vi "Config Drive Module Get-Set.vi"(4 "Start with Default":bool, 6 "Get(f) Set(t)":bool, 7 "Set Drive Config":T1={"Drive HW Ver"=0, "SparkMax Output"={"Idle Mode"=enum."Coast", "Ramp Rate (S)"=1.0}, "Slot 0 CL"={"Gains"={"P"=0.1, "I"=0.0, "D"=0.0, "F"=0.0}, "I Zone"=0.0, "Peak Out -1 0 1"={"High"=0.0, "Low"=0.0}, "Max I Accu"=0.0}, "Slot 0 SM"={"Max Velocity"=0.0, "Max Acceleration"=0.0, "Allowed CL Error"=0.0, "Min Velocity Output"=0.0}} {"Slot 0 CL"."Gains"."F" format="%#.8f"; "Slot 0 CL"."Gains"."D" format="%#.8f"; "Slot 0 CL"."Gains"."I" format="%#.8f"; "Slot 0 CL"."Gains"."P" format="%#.8f"; "Slot 0 CL"."Peak Out -1 0 1"."Low" format="%#.8f"; "Slot 0 CL"."Peak Out -1 0 1"."High" format="%#.8f"}, 8 "Error":errorcluster, 11 "Drive Refs":T8) -> (0 "Error Out":errorcluster, 3 "Drive Refs Out":T8, 5 "Drive Config Out":T1={"Drive HW Ver"=0, "SparkMax Output"={"Idle Mode"=enum."Coast", "Ramp Rate (S)"=1.0}, "Slot 0 CL"={"Gains"={"P"=0.1, "I"=0.0, "D"=0.0, "F"=0.0}, "I Zone"=0.0, "Peak Out -1 0 1"={"High"=0.0, "Low"=0.0}, "Max I Accu"=0.0}, "Slot 0 SM"={"Max Velocity"=0.0, "Max Acceleration"=0.0, "Allowed CL Error"=0.0, "Min Velocity Output"=0.0}} {"Slot 0 CL"."Gains"."F" format="%#.8f"; "Slot 0 CL"."Gains"."D" format="%#.8f"; "Slot 0 CL"."Gains"."I" format="%#.8f"; "Slot 0 CL"."Gains"."P" format="%#.8f"; "Slot 0 CL"."Peak Out -1 0 1"."Low" format="%#.8f"; "Slot 0 CL"."Peak Out -1 0 1"."High" format="%#.8f"})   [LabVIEW 2023, in "Swerve AM_ACT.lvlib"]
uses:
  Swerve AM_ACT.lvlib
  t-shirt-robot/T-Shirt Robot LV 2020/roboRIO Code/Systems/SwerveDrive AM/Cluster_Config Drive HW Values.ctl
  Shared Code/TypeDefs/Cluster_Config Spark Max Motor Output.ctl
  <vilib>/Rock Robotics/WPI/ThirdParty/REV Robotics/REVLib/Typedef/Spark MAX Idle Mode.ctl
  Shared Code/TypeDefs/Cluster_Spark MAX SLOT PID Config.ctl
  Shared Code/TypeDefs/Cluster_PID Gains.ctl
  Shared Code/TypeDefs/Cluster_High-Low.ctl
  Shared Code/TypeDefs/Cluster_SparkMax Smart Motion Parameters.ctl
  <vilib>/Rock Robotics/WPI/MotorControl/WPI_MotorControlDeviceRef.ctl
  <vilib>/Rock Robotics/WPI/MotorControl/WPI_MotorControlType.ctl
  <vilib>/Rock Robotics/SystemInterfaces/DIO/FPGA_DIOPWMChannel.ctl
  <vilib>/Rock Robotics/WPI/PWM/WPI_PWMDeadband.ctl
  <vilib>/Rock Robotics/SystemInterfaces/DIO/FPGA_DIOChannel.ctl
  <vilib>/Utility/error.llb/Trim Whitespace One-Sided.vi
  <vilib>/Utility/Data Type/NI_Data Type.lvlib
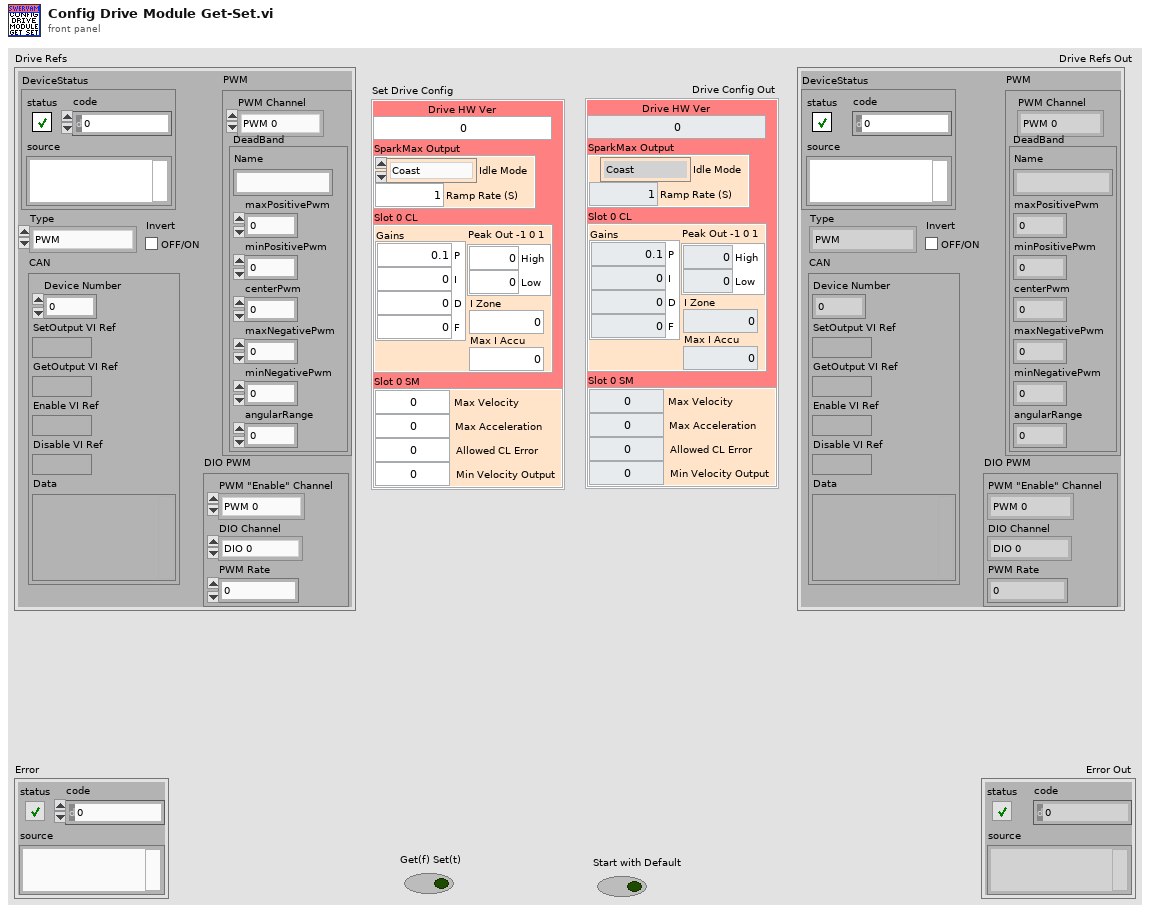
[diagram p1: front panel]
types:
  T1 = typedef "Swerve AM_ACT.lvlib/Cluster_Config Drive HW Values.ctl" = cluster{"Drive HW Ver":u64, "SparkMax Output":T2, "Slot 0 CL":T4, "Slot 0 SM":T7}
  T2 = typedef "Cluster_Config Spark Max Motor Output.ctl" = cluster{"Idle Mode":T3, "Ramp Rate (S)":dbl}
  T3 = typedef "Spark MAX Idle Mode.ctl" = enum16{"Coast", "Brake"}
  T4 = typedef "Cluster_Spark MAX SLOT PID Config.ctl" = cluster{"Gains":T5, "I Zone":dbl, "Peak Out -1 0 1":T6, "Max I Accu":dbl}
  T5 = typedef "Cluster_PID Gains.ctl" = cluster{"P":dbl, "I":dbl, "D":dbl, "F":dbl}
  T6 = typedef "Cluster_High-Low.ctl" = cluster{"High":dbl, "Low":dbl}
  T7 = typedef "Cluster_SparkMax Smart Motion Parameters.ctl" = cluster{"Max Velocity":dbl, "Max Acceleration":dbl, "Allowed CL Error":dbl, "Min Velocity Output":dbl}
  T8 = typedef "WPI_MotorControlDeviceRef.ctl" = cluster{"DeviceStatus":errorcluster, "Type":T9, "PWM":cluster{"PWM Channel":T10, "DeadBand":T11}, "CAN":cluster{"Device Number":u8, "SetOutput VI Ref":variant, "GetOutput VI Ref":variant, "Enable VI Ref":variant, "Disable VI Ref":variant, "Data":variant}, "Invert":bool, "DIO PWM":cluster{"PWM \"Enable\" Channel":T10, "DIOChannel":T12, "PWM Rate":dbl}}
  T9 = typedef "WPI_MotorControlType.ctl" = enum16{"PWM", "CAN", "DIO PWM"}
  T10 = typedef "FPGA_DIOPWMChannel.ctl" = enum8{"PWM 0", "PWM 1", "PWM 2", "PWM 3", "PWM 4", "PWM 5", "PWM 6", "PWM 7", "PWM 8", "PWM 9", "PWM MXP 0", "PWM MXP 1", "PWM MXP 2", "PWM MXP 3", "PWM MXP 4", "PWM MXP 5", "PWM MXP 6", "PWM MXP 7", "PWM MXP 8", "PWM MXP 9", "Invalid"}
  T11 = typedef "WPI_PWMDeadband.ctl" = cluster{"Name":string, "maxPositivePwm":i32, "minPositivePwm":i32, "centerPwm":i32, "maxNegativePwm":i32, "minNegativePwm":i32, "angularRange":u16}
  T12 = typedef "FPGA_DIOChannel.ctl" = enum8{"DIO 0", "DIO 1", "DIO 2", "DIO 3", "DIO 4", "DIO 5", "DIO 6", "DIO 7", "DIO 8", "DIO 9", "DIO MXP 0", "DIO MXP 1", "DIO MXP 2", "DIO MXP 3", "DIO MXP 4", "DIO MXP 5", "DIO MXP 6", "DIO MXP 7", "DIO MXP 8", "DIO MXP 9", "DIO MXP 10", "DIO MXP 11", "DIO MXP 12", "DIO MXP 13", "DIO MXP 14", "DIO MXP 15", "SPI Port CS1", "SPI Port CS2", "SPI Port CS3", "SPI Port MISO", "SPI Port MOSI", "Invalid"}
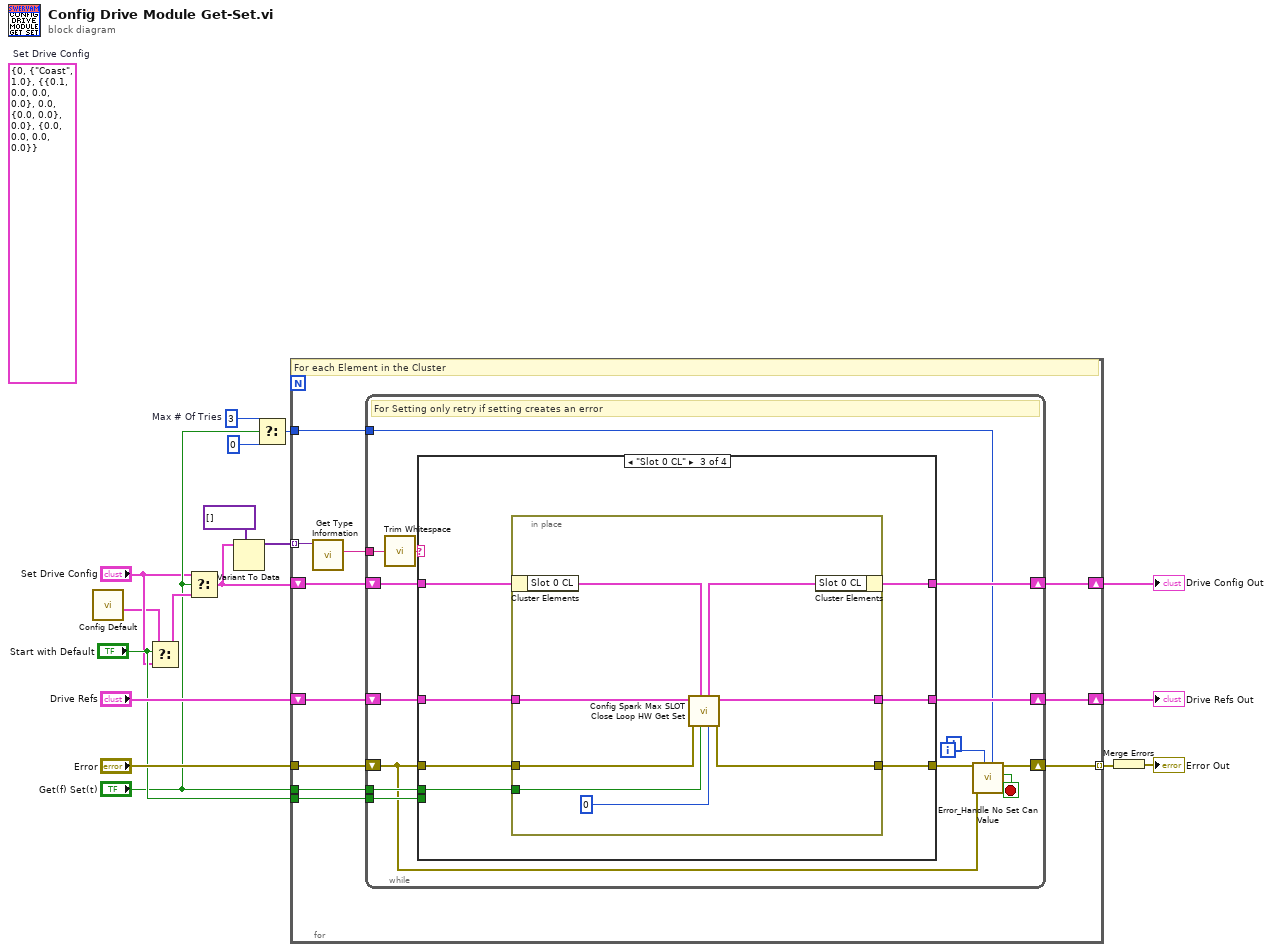
[diagram p0: block diagram]
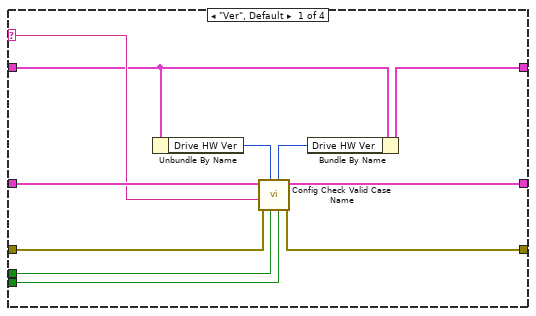
[diagram p2: hidden frame]
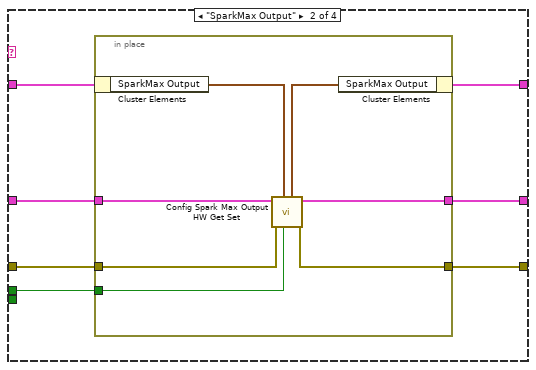
[diagram p3: hidden frame]
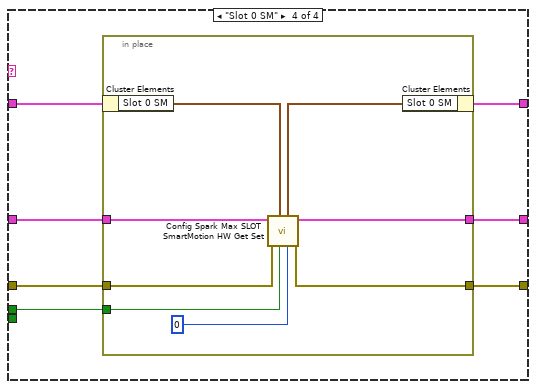
[diagram p4: hidden frame]
diagram:
  w5 = 3  # Max # Of Tries
  (unwired) T1 {"Drive HW Ver"=0, "SparkMax Output"={"Idle Mode"=enum."Coast", "Ramp Rate (S)"=1.0}, "Slot 0 CL"={"Gains"={"P"=0.1, "I"=0.0, "D"=0.0, "F"=0.0}, "I Zone"=0.0, "Peak Out -1 0 1"={"High"=0.0, "Low"=0.0}, "Max I Accu"=0.0}, "Slot 0 SM"={"Max Velocity"=0.0, "Max Acceleration"=0.0, "Allowed CL Error"=0.0, "Min Velocity Output"=0.0}}  # Set Drive Config
  n1 = call "Config Default.vi"() -> ("Drive Default Out"=w1:T1)  [unwired: 8 in, 3 out]
  n2 = Select(t=w1, s="Start with Default", f="Set Drive Config") -> (s? t:f=w8:T1)
  n3 = Select(t="Set Drive Config", s="Get(f) Set(t)", f=w8) -> (s? t:f=w9:T1)
  n4 = Variant To Data(type=variant[] [], Variant=w9) -> (data=w15:variant[])  [unwired: 1 in, 1 out]
  n5 = Select(t=w5, s="Get(f) Set(t)", f=0) -> (s? t:f=w3:i32)
  n6 = for {
    tunnel: w15 -> [w27] mode=indexing
    shift-right: [w24] -> w14
    shift-left: w9 -> [w25]
    tunnel: "Error" -> [w23]
    tunnel: [w22] -> w13 mode=indexing
    shift-right: [w21] -> w10
    shift-left: "Drive Refs" -> [w26]
    tunnel: "Get(f) Set(t)" -> [w20]
    tunnel: "Start with Default" -> [w19]
    tunnel: w3 -> [w18]
    # "For each Element in the Cluster"
    n7 = call <vilib>:"Get Type Information.vi"("variant"=w27) -> ("name"=w28:string)  [unwired: 6 in, 4 out]
    n8 = while {
      tunnel: w28 -> [w42]
      tunnel: w20 -> [w36]
      tunnel: w19 -> [w35]
      shift-right: [w37] -> w21
      shift-left: w26 -> [w40]
      shift-right: [w38] -> w24
      shift-left: w25 -> [w39]
      shift-right: [w33] -> w22
      shift-left: w23 -> [w32]
      tunnel: w18 -> [w30]
      i -> [w31]
      stop <- w29 stop-if-true
      # "For Setting only retry if setting creates an error"
      n9 = call <vilib>:"Trim Whitespace.vi"("string"=w42) -> ("trimmed string"=w41:string)  [unwired: 1 in]
      n10 = case shown="\"Slot 0 CL\"" w41 {
        selector: w41 -> [w49 _ _ _]
        tunnel: w40 -> [w53 w58 w72 w87]
        tunnel: w39 -> [w45 w60 w74 w89]
        tunnel: [w44 w59 w73 w88] -> w38
        tunnel: w32 -> [w51 w56 w70 w85]
        tunnel: [w50 w55 w69 w84] -> w34
        tunnel: [w52 w57 w71 w86] -> w37
        tunnel: w36 -> [w48 w54 w68 w83]
        tunnel: w35 -> [w47 _ _ _]
        frame "Ver", Default {
          n11 = Unbundle By Name(w45) -> ("Drive HW Ver"=w46:u64)
          n12 = call "Config Check Valid Case Name.vi"("Start With Default"=w47, "Get(f) Set(t)"=w48, "Ver"=w46, "Error"=w51, "Case Name"=w49, "Steer Refs"=w53) -> ("Error Out"=w50:errorcluster, "Steer Refs Out"=w52:T8, "Ver Out"=w43:u64)  [unwired: 3 in]
          n13 = Bundle By Name(cluster=w45, "Drive HW Ver"=w43) -> (w44:T1)
        }
        frame "SparkMax Output" {
          n14 = in-place {
            in-place-border: w58 -> [w63]
            in-place-border: [w62] -> w57
            in-place-border: w56 -> [w67]
            in-place-border: [w66] -> w55
            in-place-border: w54 -> [w61]
            n15 = in-place-cluster #1(w60) -> ("SparkMax Output"=w65:T2)
            n16 = call "Config Spark Max Output HW Get Set.vi"("Get(f) Set(t)"=w61, "SparkMax Output"=w65, "Error"=w67, "Drive Refs"=w63) -> ("Error Out"=w66:errorcluster, "Drive Refs Out"=w62:T8, "SparkMax Output Out"=w64:T2)  [unwired: 5 in]
            n17 = in-place-cluster #1("SparkMax Output"=w64) -> (w59:T1)
          }
        }
        frame "Slot 0 CL" {
          n18 = in-place {
            in-place-border: w72 -> [w78]
            in-place-border: [w77] -> w71
            in-place-border: w70 -> [w82]
            in-place-border: [w81] -> w69
            in-place-border: w68 -> [w76]
            n19 = in-place-cluster #2(w74) -> ("Slot 0 CL"=w80:T4)
            n20 = call "Config Spark Max SLOT Close Loop HW Get Set.vi"("PIDF Slot (0)"=0, "Get(f) Set(t)"=w76, "SparkMax Slot CL"=w80, "Error"=w82, "Drive Refs"=w78) -> ("Error Out"=w81:errorcluster, "Drive Refs Out"=w77:T8, "SparkMax Slot CL Out"=w79:T4)  [unwired: 4 in]
            n21 = in-place-cluster #2("Slot 0 CL"=w79) -> (w73:T1)
          }
        }
        frame "Slot 0 SM" {
          n22 = in-place {
            in-place-border: w87 -> [w94]
            in-place-border: [w95] -> w86
            in-place-border: w85 -> [w93]
            in-place-border: [w92] -> w84
            in-place-border: w83 -> [w90]
            n23 = in-place-cluster #3(w89) -> ("Slot 0 SM"=w97:T7)
            n24 = call "Config Spark Max SLOT SmartMotion HW Get Set.vi"("PIDF Slot (0)"=0, "Get(f) Set(t)"=w90, "SparkMax Slot SM"=w97, "Error"=w93, "Drive Refs"=w94) -> ("Error Out"=w92:errorcluster, "Drive Refs Out"=w95:T8, "SparkMax Slot SM Out"=w96:T7)  [unwired: 4 in]
            n25 = in-place-cluster #3("Slot 0 SM"=w96) -> (w88:T1)
          }
        }
      }
      n26 = call "Error_Handle No Set Can Value.vi"("Max # Of Tries"=w30, "Loop Itteration"=w31, "Previous Error"=w32, "Error"=w34) -> ("Stop Out"=w29:bool, "Error Out"=w33:errorcluster)  [unwired: 6 in]
    }
  }
  "Drive Refs Out" <- w10
  "Drive Config Out" <- w14
  n27 = Merge Errors(w13) -> (→"Error Out":errorcluster)
